vi "Set Manual wrapper.vi"(1 "Manual":bool, 2 "PIDClass string":string) -> (0 "PIDClass string out":string)   [LabVIEW 2013]
uses:
  PIDClass.lvclass
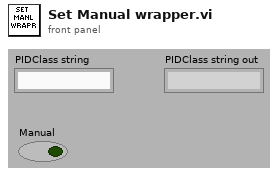
[diagram p1: front panel]
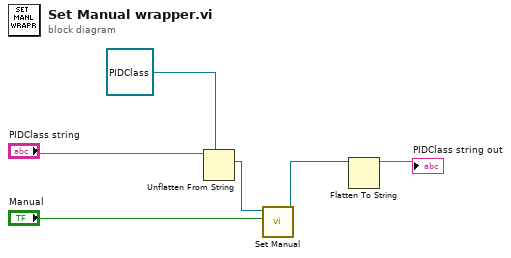
[diagram p0: block diagram]
diagram:
  n1 = Unflatten From String(type=refnum<class "PIDClass.lvclass"> refnum ("PIDClass.lvclass out"), binary string="PIDClass string") -> (value=w3:refnum<class "PIDClass.lvclass">)  [unwired: 1 in, 4 out]
  n2 = call "Set Manual.vi"("Manual"="Manual", "PIDClass.lvclass"=w3) -> ("PIDClass.lvclass out"=w5:refnum<class "PIDClass.lvclass">)  [unwired: 9 out]
  n3 = Flatten To String(anything=w5) -> (data string=→"PIDClass string out":string)  [unwired: 1 in, 4 out]
